vi "Teleop.vi"(8 "State Machine In":enum16{"Scale", "Switch", "Intake", "Reserve"}(ring), 10 "Match Info":T1={"Autonomous Elapsed Seconds"=0.0, "TeleOp Elapsed Seconds"=0.0, "Disabled Elapsed Seconds"=0.0, "Visited Autonomous"=FALSE, "Visited TeleOp"=FALSE, "Visited Disabled"=FALSE, "Autonomous Settings"={"Autonomous Style"=enum."Independent", "VI Refnum"=refnum}}, 11 "Call Context":T2) -> (0 "State Machine Out":enum16{"Scale", "Switch", "Intake", "Reserve"}(ring))   [LabVIEW 2018]
doc: "This VI is called for each enabled TeleOp packet received from the DS. It is typically used to read from joysticks and other inputs and update I/O or setpoints for timed control loops. It should complete and return within 20 milliseconds or risk missing DS packets."
uses:
  <vilib>/Rock Robotics/WPI/DriverStation/WPI_DriverStationDerivedRobotMode.ctl
  <vilib>/Rock Robotics/WPI/DriverStation/WPI_DriverStationMatch Info.ctl
  <vilib>/Rock Robotics/WPI/Utilities/WPI_GetSetVariantRefNum.vi
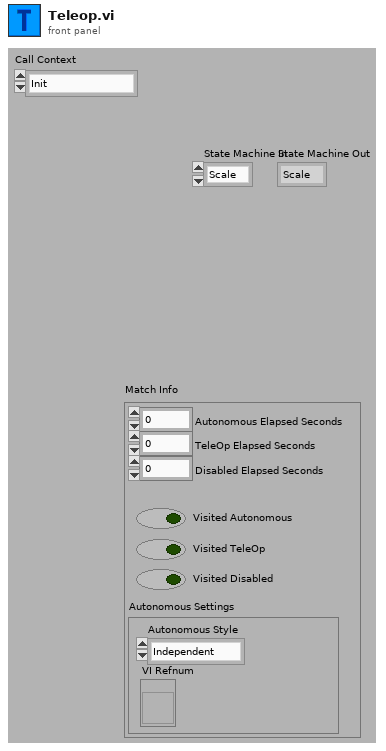
[diagram p1: front panel]
types:
  T1 = typedef "WPI_DriverStationMatch Info.ctl" = cluster{"Autonomous Elapsed Seconds":dbl, "TeleOp Elapsed Seconds":dbl, "Disabled Elapsed Seconds":dbl, "Visited Autonomous":bool, "Visited TeleOp":bool, "Visited Disabled":bool, "Autonomous Settings":cluster{"Autonomous Style":enum16{"Iterative", "Independent"}, "VI Refnum":refnum<vi>}}
  T2 = typedef "WPI_DriverStationDerivedRobotMode.ctl" = enum16{"Init", "Execute", "Stop"}
  T3 = typedef "WPI_JoystickDevRef.ctl" = cluster{"Device":T4}
  T4 = typedef "WPI_JoystickDeviceEnum.ctl" = enum16{"USB 0", "USB 1", "USB 2", "USB 3", "USB 4", "USB 5"}
  T5 = cluster{"POVs[0]":i16, "POVs[1]":i16, "POVs[2]":i16, "POVs[3]":i16, "POVs[4]":i16, "POVs[5]":i16, "POVs[6]":i16, "POVs[7]":i16, "POVs[8]":i16}
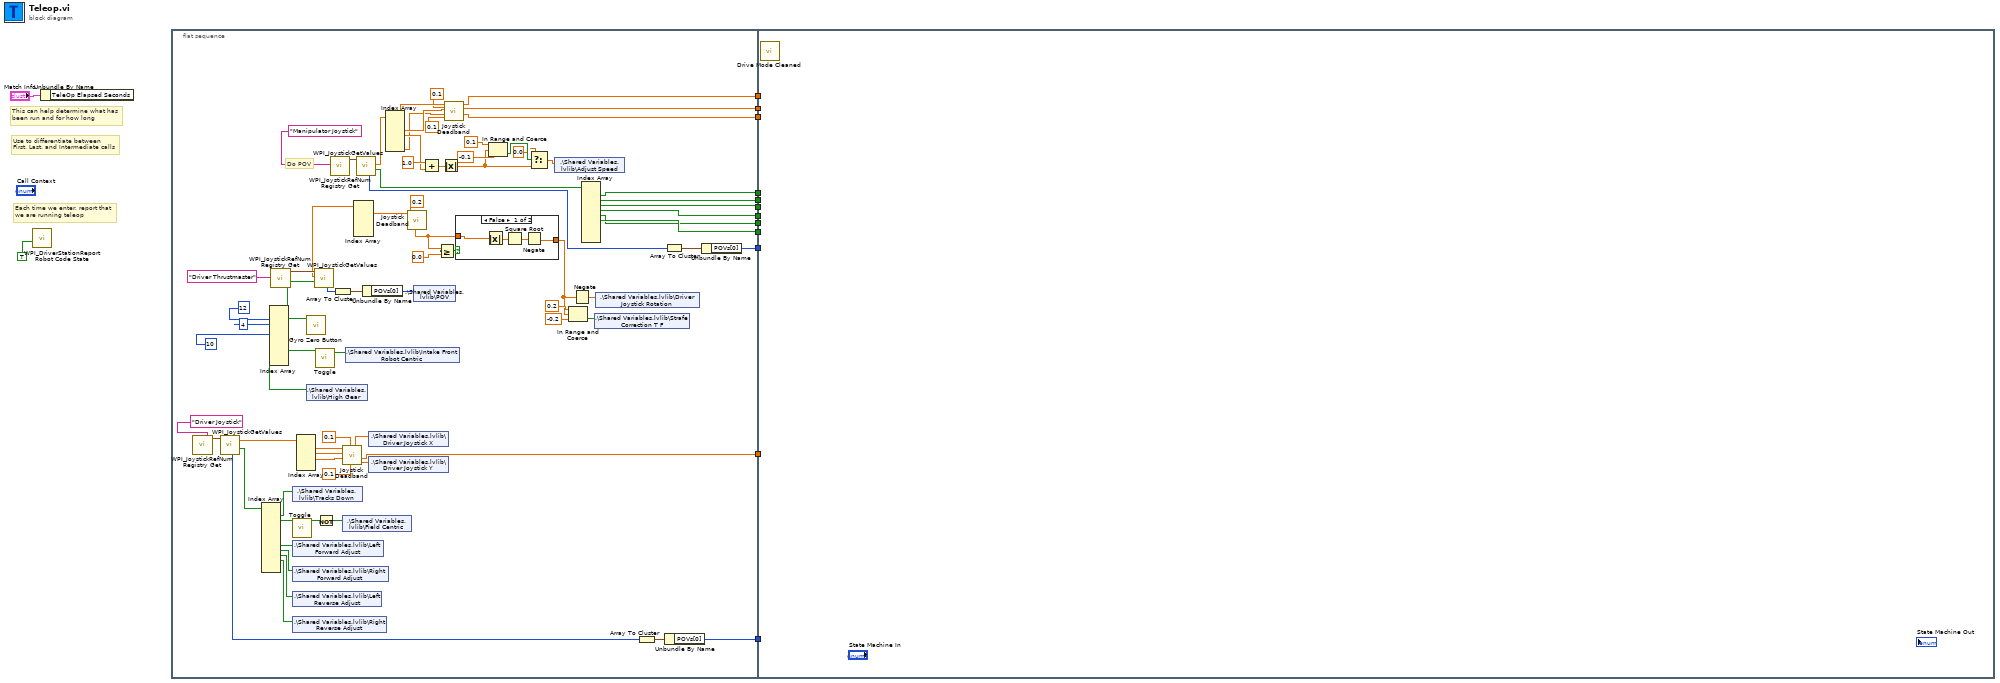
[diagram p0: block diagram]
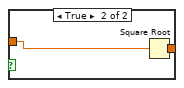
[diagram p2: hidden frame]
diagram:
  # "Each time we enter, report that\nwe are running teleop"
  # "Use to differentiate between\nFirst, Last, and Intermediate calls"
  # "This can help determine what has\nbeen run and for how long"
  n1 = call <vilib>:"WPI_DriverStationReport Robot Code State.vi"("TeleOp"=TRUE ("Autonomous")) -> ()  [unwired: 10 in, 1 out]
  n2 = Unbundle By Name("Match Info") -> ()  [unwired: 1 out]
  n3 = flat-sequence {
    tunnel: [w48] -> w12
    tunnel: [w38] -> w11
    tunnel: [w35] -> w10
    tunnel: [w34] -> w9
    tunnel: [w40] -> w8
    tunnel: [w39] -> w7
    tunnel: [w43] -> w6
    tunnel: [w42] -> w5
    tunnel: [w41] -> w4
    tunnel: [w30] -> w3
    tunnel: [w29] -> w2
    tunnel: [w17] -> w1
    tunnel: w12 -> [_]
    tunnel: w11 -> [_]
    tunnel: w10 -> [_]
    tunnel: w9 -> [_]
    tunnel: w8 -> [_]
    tunnel: w7 -> [_]
    tunnel: w6 -> [_]
    tunnel: w5 -> [_]
    tunnel: w4 -> [_]
    tunnel: w3 -> [_]
    tunnel: w2 -> [_]
    tunnel: w1 -> [_]
    frame #0 {
      # "Do POV"
      n4 = call <vilib>:"WPI_JoystickRefNum Registry Get.vi"("refnum name"="Driver Joystick") -> ("JoystickDevRef"=w91:T3)  [unwired: 1 in, 9 out]
      n5 = call <vilib>:"WPI_JoystickGetValues.vi"("JoystickDevRef"=w91) -> ("Buttons"=w68:bool[], "Axes"=w89:dbl[], "POVs"=w49:i16[])  [unwired: 6 in, 2 out]
      n6 = Index Array(array=w68) -> (element #1=w16:bool, element #2=w15:bool, element #7=w28:bool, element #8=w27:bool, element #9=w26:bool, element #10=w25:bool)  [unwired: 12 in, 6 out]
      n7 = call <vilib>:"WPI_JoystickRefNum Registry Get.vi"("refnum name"="Driver Thrustmaster") -> ("JoystickDevRef"=w78:T3)  [unwired: 9 in, 1 out]
      n8 = shared-variable ".\\Shared Variables.lvlib\\Tracks Down"(w16) -> ()  [unwired: 1 in, 1 out]
      n9 = call "Toggle.vi"("Input"=w15) -> ("Output"=w84:bool)  [unwired: 9 in, 1 out]
      n10 = shared-variable ".\\Shared Variables.lvlib\\Left Forward Adjust"(w28) -> ()  [unwired: 1 in, 1 out]
      n11 = shared-variable ".\\Shared Variables.lvlib\\Right Forward Adjust"(w27) -> ()  [unwired: 1 in, 1 out]
      n12 = shared-variable ".\\Shared Variables.lvlib\\Left Reverse Adjust"(w26) -> ()  [unwired: 1 in, 1 out]
      n13 = shared-variable ".\\Shared Variables.lvlib\\Right Reverse Adjust"(w25) -> ()  [unwired: 1 in, 1 out]
      n14 = Index Array(array=w89) -> (element #1=w82:dbl, element #2=w81:dbl, element #4=w18:dbl)  [unwired: 5 in, 2 out]
      n15 = call <vilib>:"WPI_JoystickGetValues.vi"("JoystickDevRef"=w78) -> ("Buttons"=w60:bool[], "Axes"=w77:dbl[], "POVs"=w51:i16[])  [unwired: 6 in, 2 out]
      n16 = Index Array(array=w60, index #1=12 ("index"), index #2=4 ("index"), index #4=10 ("index")) -> (element #1=w58:bool, element #2=w33:bool, element #4=w52:bool)  [unwired: 7 in, 7 out]
      n17 = call "Gyro Zero Button.vi"("Boolean"=w58) -> ()  [unwired: 11 in]
      n18 = shared-variable ".\\Shared Variables.lvlib\\High Gear"(w33) -> ()  [unwired: 1 in, 1 out]
      n19 = call "Toggle.vi"("Input"=w52) -> ("Output"=w53:bool)  [unwired: 9 in, 1 out]
      n20 = Not(x=w84) -> (.not. x?=w80:bool)
      n21 = call <vilib>:"WPI_JoystickRefNum Registry Get.vi"("refnum name"="Manipulator Joystick") -> ("JoystickDevRef"=w87:T3)  [unwired: 1 in, 9 out]
      n22 = Array To Cluster(array=w51) -> (cluster=w56:T5)
      n23 = call "Joystick Deadband.vi"("Z Deadband"=0.1, "X Y Deadband"=0.1, "Z"=w18, "Y"=w81, "X"=w82) -> ("Z Out"=w17:dbl, "Y Out"=w85:dbl, "X Out"=w23:dbl)  [unwired: 4 in]
      n24 = shared-variable ".\\Shared Variables.lvlib\\Field Centric"(w80) -> ()  [unwired: 1 in, 1 out]
      n25 = shared-variable ".\\Shared Variables.lvlib\\Intake Front Robot Centric"(w53) -> ()  [unwired: 1 in, 1 out]
      n26 = Index Array(array=w77) -> (element #1=w22:dbl)  [unwired: 5 in, 4 out]
      n27 = call <vilib>:"WPI_JoystickGetValues.vi"("JoystickDevRef"=w87) -> ("Buttons"=w83:bool[], "Axes"=w73:dbl[], "POVs"=w31:i16[])  [unwired: 6 in, 2 out]
      n28 = Unbundle By Name(w56) -> ("POVs[0]"=w55:i16)
      n29 = shared-variable ".\\Shared Variables.lvlib\\Driver Joystick X"(w23) -> ()  [unwired: 1 in, 1 out]
      n30 = shared-variable ".\\Shared Variables.lvlib\\Driver Joystick Y"(w85) -> ()  [unwired: 1 in, 1 out]
      n31 = Index Array(array=w73) -> (element #1=w46:dbl, element #2=w37:dbl, element #3=w64:dbl, element #6=w36:dbl)  [unwired: 6 in, 2 out]
      n32 = call "Joystick Deadband.vi"("X Y Deadband"=0.2, "X"=w22) -> ("X Out"=w20:dbl)  [unwired: 7 in, 2 out]
      n33 = shared-variable ".\\Shared Variables.lvlib\\POV"(w55) -> ()  [unwired: 1 in, 1 out]
      n34 = Add(x=1.0, y=w64) -> (x+y=w67:dbl)
      n35 = Greater Or Equal?(x=w20, y=0.0) -> (x >= y?=w63:bool)
      n36 = Absolute Value(x=w67) -> (abs(x)=w65:dbl)
      n37 = call "Joystick Deadband.vi"("Z Deadband"=0.1, "X Y Deadband"=0.1, "Z"=w36, "Y"=w37, "X"=w46) -> ("Z Out"=w34:dbl, "Y Out"=w35:dbl, "X Out"=w38:dbl)  [unwired: 4 in]
      n38 = case shown="False" w63 {
        tunnel: [w93 w97] -> w19
        tunnel: w20 -> [w92 w96]
        frame False {
          n39 = Absolute Value(x=w92) -> (abs(x)=w95:dbl)
          n40 = Square Root(x=w95) -> (sqrt(x)=w94:dbl)
          n41 = Negate(x=w94) -> (-x=w93:dbl)
        }
        frame True {
          n42 = Square Root(x=w96) -> (sqrt(x)=w97:dbl)
        }
      }
      n43 = In Range and Coerce(upper limit=0.1, x=w65, lower limit=-0.1 ("x")) -> (In Range?=w70:bool)  [unwired: 1 out]
      n44 = Select(t=0.0, s=w70, f=w65) -> (s? t:f=w61:dbl)
      n45 = shared-variable ".\\Shared Variables.lvlib\\Adjust Speed"(w61) -> ()  [unwired: 1 in, 1 out]
      n46 = In Range and Coerce(upper limit=0.2, x=w19, lower limit=-0.2) -> (In Range?=w76:bool)  [unwired: 1 out]
      n47 = Negate(x=w19) -> (-x=w24:dbl)
      n48 = Index Array(array=w83) -> (element #1=w41:bool, element #2=w40:bool, element #3=w39:bool, element #4=w42:bool, element #5=w29:bool, element #6=w43:bool)  [unwired: 10 in, 4 out]
      n49 = shared-variable ".\\Shared Variables.lvlib\\Strafe Correction T F"(w76) -> ()  [unwired: 1 in, 1 out]
      n50 = shared-variable ".\\Shared Variables.lvlib\\Driver Joystick Rotation"(w24) -> ()  [unwired: 1 in, 1 out]
      n51 = Array To Cluster(array=w49) -> (cluster=w50:T5)
      n52 = Array To Cluster(array=w31) -> (cluster=w32:T5)
      n53 = Unbundle By Name(w50) -> ("POVs[0]"=w48:i16)
      n54 = Unbundle By Name(w32) -> ("POVs[0]"=w30:i16)
    }
    frame #1 {
      n55 = call "Drive Mode Cleaned.vi"() -> ()  [unwired: 12 in]
    }
  }
